vi "Email Testing.vi"() -> ()   [LabVIEW 2019]
uses:
  <vilib>/regexp/Match Regular Expression.xnode
panel:
  out "output":string[](array[string])
  out "error":string[](array[string])
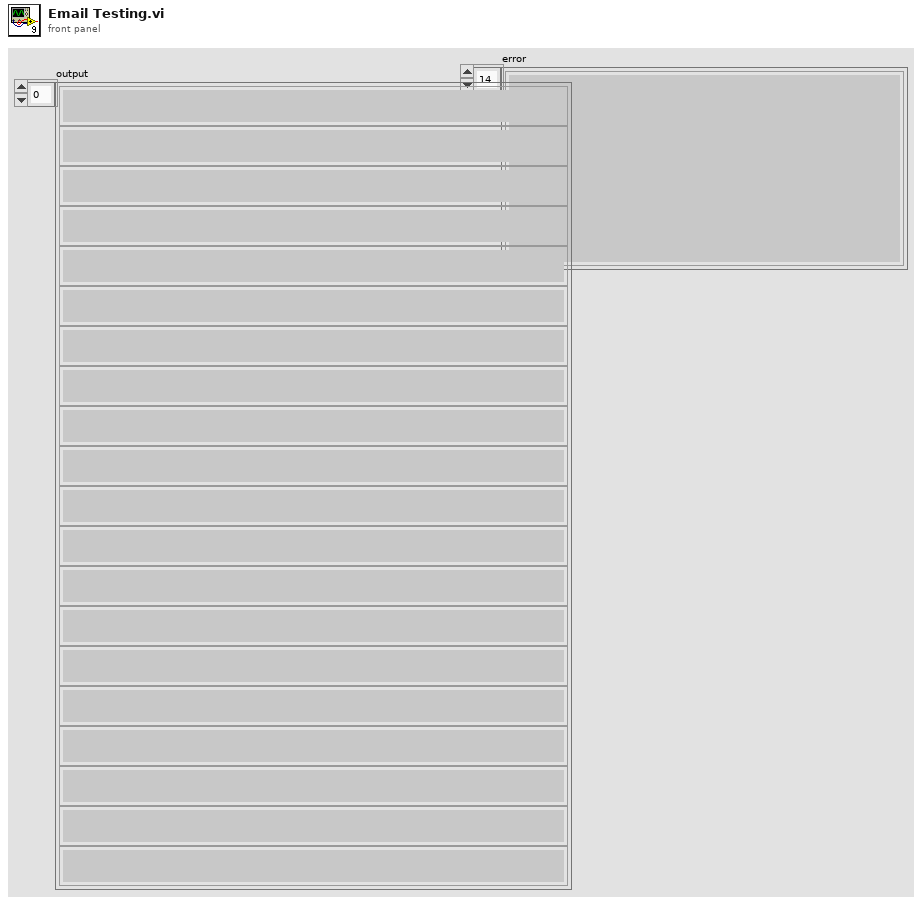
[diagram p1: front panel]
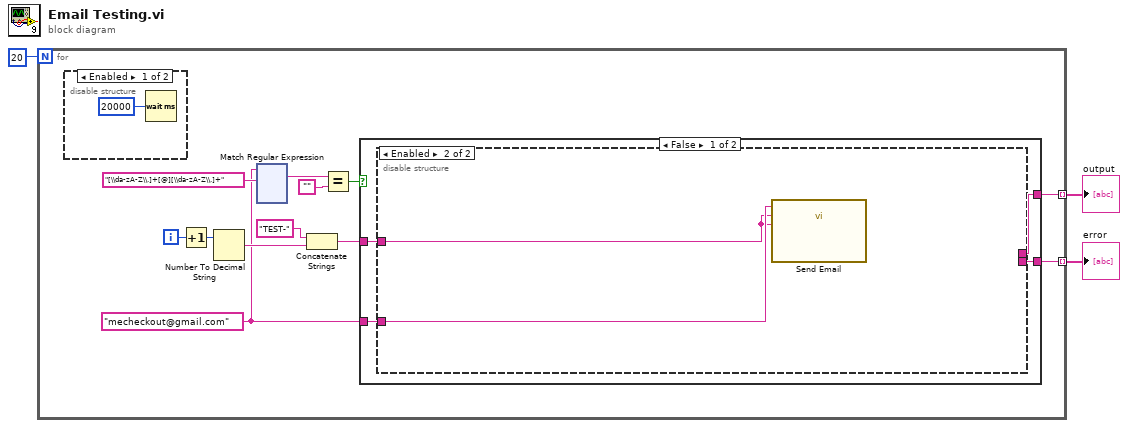
[diagram p0: block diagram]
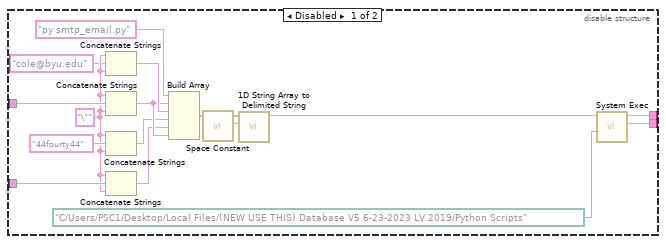
[diagram p3: hidden frame]
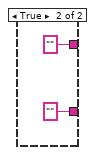
[diagram p4: hidden frame]
diagram:
  n1 = for {
    N: 20 -> [_]
    tunnel: [w7] -> w2 mode=indexing
    tunnel: [w6] -> w1 mode=indexing
    i -> [w4]
    w8 = "mecheckout@gmail.com" ("input string")
    n2 = disable-structure shown="Enabled" {
      frame Enabled {
        n3 = Wait (ms)(milliseconds to wait=u32 20000) -> ()  [unwired: 1 out]
      }
      frame Disabled {
      }
    }
    n4 = Increment(x=w4) -> (x+1=w5:i32)
    n5 = Number To Decimal String(number=w5) -> (decimal integer string=w10:string)  [unwired: 1 in]
    n6 = xnode "Match Regular Expression"("input string"=w8, "regular expression"="[\\da-zA-Z\\.]+[@][\\da-zA-Z\\.]+" ("search string")) -> ("whole match"=w14:string)  [unwired: 4 in, 4 out]
    n7 = Concatenate Strings("TEST-", w10) -> (w9:string)
    n8 = Equal?(x=w14, y="") -> (x = y?=w15:bool)
    n9 = case shown="False" w15 {
      tunnel: w8 -> [w134 _]
      tunnel: w9 -> [w133 _]
      tunnel: [w132 "" ("standard error")] -> w7
      tunnel: [w131 "" ("standard output")] -> w6
      frame False {
        n10 = disable-structure shown="Enabled" {
          disable-tunnel: w134 -> [w148 w152]
          disable-tunnel: w133 -> [w147 w151]
          disable-tunnel: [w136 _] -> w132
          disable-tunnel: [w135 _] -> w131
          frame Disabled {
            w145 = "\""
            n11 = Concatenate Strings(w145, "cole@byu.edu" ("string"), w145) -> (w143:string)
            n12 = Concatenate Strings(w145, w147, w145) -> (w142:string)
            n13 = Concatenate Strings(w145, "44fourty44" ("string"), w145) -> (w141:string)
            n14 = Concatenate Strings(w145, w148, w145) -> (w140:string)
            n15 = Build Array("py smtp_email.py", w142, w143, w141, w140, w142) -> (w139:string[])
            n16 = call <vilib>:"Space Constant.vi"() -> ("String"=w138:string)
            n17 = call <vilib>:"1D String Array to Delimited String.vi"("delimiter"=w138, "string array"=w139) -> ("delimited string"=w137:string)  [unwired: 9 in]
            n18 = call <vilib>:"System Exec.vi"("working directory"=path "C:/Users/PSC1/Desktop/Local Files/(NEW USE THIS) Database V5 6-23-2023 LV 2019/Python Scripts", "command line"=w137) -> ("standard error"=w136:string, "standard output"=w135:string)  [unwired: 6 in, 2 out]
          }
          frame Enabled {
            n19 = call "Send Email"("Message"=w151, "Subject"=w151, "Recipients"=w152) -> ()  [unwired: 8 in, 1 out]
          }
        }
      }
      frame True {
      }
    }
  }
  "error" <- w2
  "output" <- w1
